vi "Handle Mouse Down.vi"(6 "Vertical Position":i32 caption="垂直位置", 8 "error in (no error)":errorcluster caption="错误输入（无错误）", 9 "Browse Dir Ref":refnum<vi> caption="浏览目录引用", 10 "Editing Path Ref":refnum<vi> caption="编辑路径引用", 11 "Include Paths Ref":refnum<vi> caption="包括路径引用") -> (0 "error out":errorcluster caption="错误输出", 1 "Row Number":i32 caption="行数")   [LabVIEW 2011, in "NISAST Include Paths.xctl"]
uses:
  NISAST Include Paths.xctl
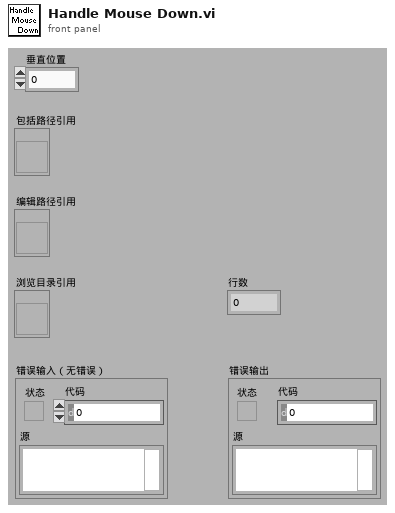
[diagram p1: front panel]
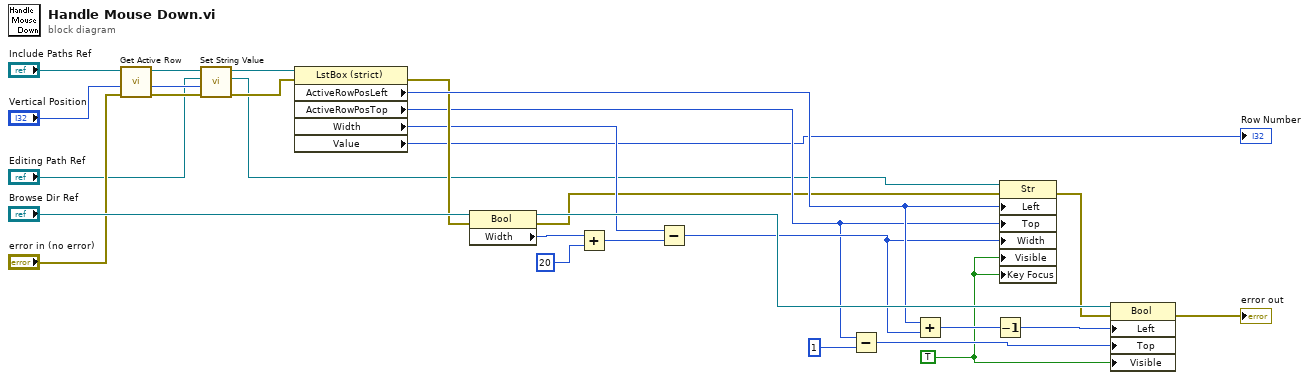
[diagram p0: block diagram]
diagram:
  w9 = TRUE ("Visible")
  n1 = call "Get Active Row.vi"("error in (no error)"="error in (no error)", "Vertical Position"="Vertical Position", "Include Paths Ref"="Include Paths Ref") -> ("error out"=w5:errorcluster, "Row Number"=w4:i32, "Dup Include Paths Ref"=w8:refnum<vi>)  [unwired: 6 in]
  n2 = call "Set String Value.vi"("error in (no error)"=w5, "Active Row Number"=w4, "Editing Path Ref"="Editing Path Ref", "Include Paths Ref"=w8) -> ("error out"=w6:errorcluster, "Dup Editing Path Ref"=w2:refnum<vi>, "Dup Include Paths Ref"=w7:refnum<vi>)  [unwired: 5 in]
  n3 = property class="LstBox (strict)"(reference=w7, error in=w6) -> (error out=w23:errorcluster, "ActiveRowPosLeft"=w25:i32, "ActiveRowPosTop"=w19:i32, "Width"=w18:u32, "Value"=→"Row Number":i32)  [unwired: 1 out]
  n4 = property class="Bool"(reference="Browse Dir Ref", error in=w23) -> (reference out=w26:refnum<vi>, error out=w1:errorcluster, "Width"=w21:u32)
  n5 = Add(x=w21, y=u32 20) -> (x+y=w20:u32)
  n6 = Subtract(x=w18, y=w20) -> (x-y=w24:u32)
  n7 = Subtract(x=w19, y=u32 1) -> (x-y=w13:u32)
  n8 = Add(x=w25, y=w24) -> (x+y=w11:u32)
  n9 = Decrement(x=w11) -> (x-1=w10:u32)
  n10 = property class="Str"(reference=w2, error in=w1, "Left"=w25, "Top"=w19, "Width"=w24, "Visible"=w9, "Key Focus"=w9) -> (error out=w14:errorcluster)  [unwired: 1 out]
  n11 = property class="Bool"(reference=w26, error in=w14, "Left"=w10, "Top"=w13, "Visible"=w9) -> (error out=→"error out":errorcluster)  [unwired: 1 out]
